vi "Information.vi"() -> (2 "Connection Info":string)   [LabVIEW 2019]
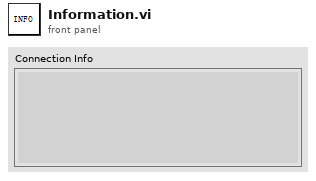
[diagram p1: front panel]
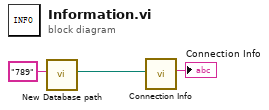
[diagram p0: block diagram]
diagram:
  n1 = call "New Database path.vi"("Database Name"="789") -> ("Database path"=w3:path)  [unwired: 10 in]
  n2 = call "Connection Info.vi"("路径"=w3) -> ("Connection Info"=→"Connection Info":string)  [unwired: 10 in]
